vi "Initialize.vi"(8 "error in (no error)":errorcluster, 11 "Image in":refnum<class "Image.lvclass">) -> (0 "error out":errorcluster, 3 "Image out":refnum<class "Image.lvclass">)   [LabVIEW 2011, in "Image.lvclass"]
uses:
  Image.lvclass
  Image.lvclass/Image.ctl
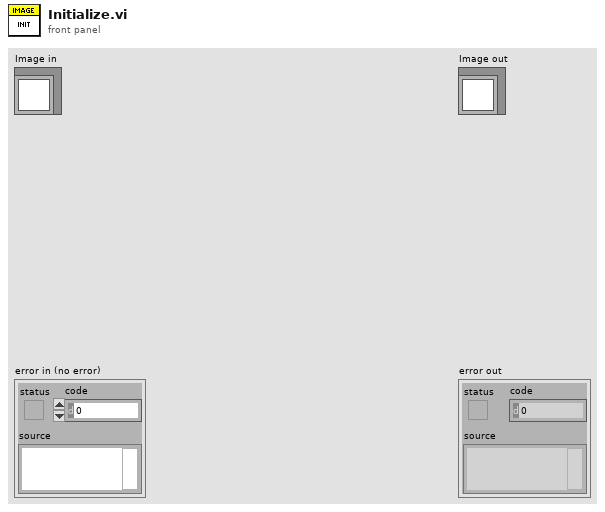
[diagram p1: front panel]
types:
  T1 = typedef "Image Type" = u32
  T2 = typedef "IMAQ Image.ctl" = refnum<image>
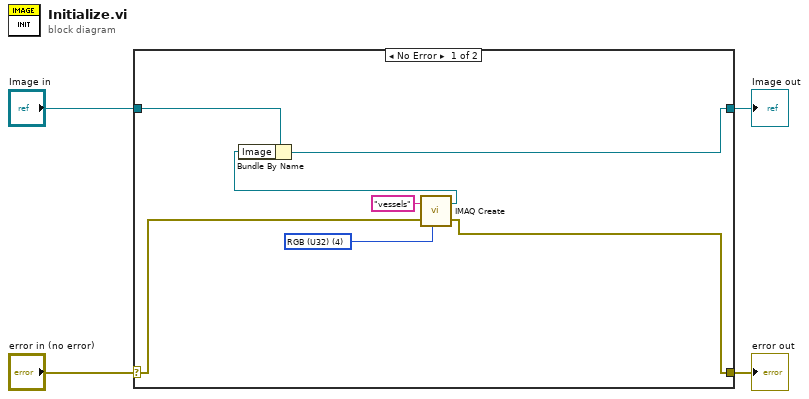
[diagram p0: block diagram]
diagram:
  n1 = case shown="No Error" "error in (no error)" {
    selector: "error in (no error)" -> [w8 w13]
    tunnel: [w7 w13] -> w3
    tunnel: [w5 w12] -> w1
    tunnel: "Image in" -> [w11 w12]
    frame No Error {
      w10 = T1 4 items=["Grayscale (U8)", "Grayscale (I16)", "Grayscale (SGL)", "Complex (CSG)", "RGB (U32)", "HSL (U32)", "RGB (U64)", "Grayscale (U16)"] ("Image Type")
      n2 = call "IMAQ Create"("Image Name"="vessels", "Image Type"=w10, "error in (no error)"=w8) -> ("New Image"=w6:T2, "error out"=w7:errorcluster)  [unwired: 2 in]
      n3 = Bundle By Name(cluster=w11, "Image"=w6) -> (w5:refnum<class "Image.lvclass">)
    }
    frame Error {
    }
  }
  "error out" <- w3
  "Image out" <- w1
